vi "TiePie.Gen.SetSignalType.vi"(8 "error in (no error)":errorcluster, 10 "signal type (sine)":u32(ring)=1 items=["sine"=1, "triangle"=2, "square"=4, "DC"=8, "noise"=16, "arbitrary"=32, "pulse"=64], 11 "GenHandle":T1) -> (0 "error out":errorcluster, 3 "GenHandle out":T1)   [LabVIEW 2014, in "LVTiePie.lvlib"]
uses:
  LVTiePie.lvlib
  TiePie.Gen.handle.ctl
  bin/libtiepie.dll
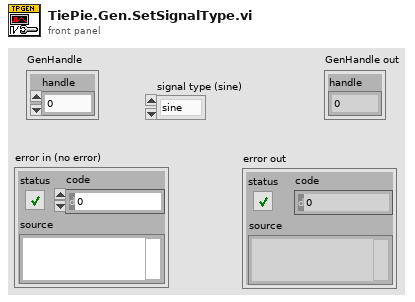
[diagram p1: front panel]
types:
  T1 = typedef "TiePie.Gen.handle.ctl" = cluster{"handle":u32}
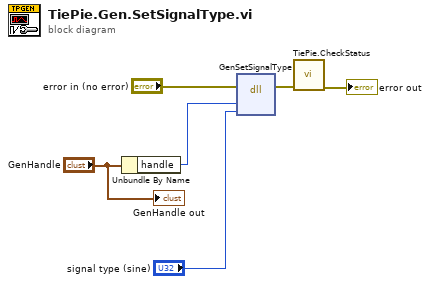
[diagram p0: block diagram]
diagram:
  n1 = Unbundle By Name("GenHandle") -> ("handle"=w5:u32)
  n2 = dll-call lib="C:/Users/mbirski/Desktop/PAN/LabVEW/Tie Pie/bin/libtiepie.dll" fn="GenSetSignalType"(error in="error in (no error)", "handle"=w5, "signal type"="signal type (sine)") -> (error out=w2:errorcluster)  [unwired: 5 in, 1 out]
  n3 = call "TiePie.CheckStatus.vi"("error in (no error)"=w2) -> ("error out"=→"error out":errorcluster)  [unwired: 10 in]
  "GenHandle out" <- "GenHandle"
